vi "read_voltage0.vi"(1 "Channel":i32 min=0 max=15) -> (0 "Voltage":dbl)   [LabVIEW 2011]
uses:
  globals.vi
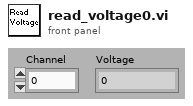
[diagram p1: front panel]
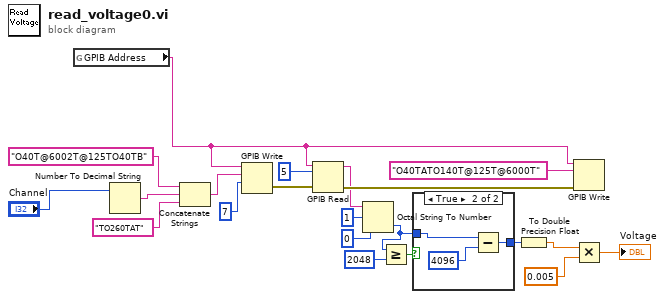
[diagram p0: block diagram]
diagram:
  n1 = global read "globals.vi" "GPIB Address"() -> (w2:string)
  n2 = Number To Decimal String(number="Channel") -> (decimal integer string=w8:string)  [unwired: 1 out]
  n3 = Concatenate Strings("O40T@6002T@125TO40TB" ("data"), w8, "TO260TAT" ("string")) -> (w7:string)
  n4 = GPIB Write(0:w2, 1:w7, 2:i16 7 ("mode (0)")) -> (6:w21:errorcluster)  [unwired: 1 in, 2 out]
  n5 = GPIB Read(0:w2, 1:5 ("byte count"), 3:w21) -> (5:w17:string, 7:w20:errorcluster)  [unwired: 3 out]
  n6 = Octal String To Number(2:0 ("default (0 U32)"), 3:1 ("offset"), 4:w17) -> (0:w11:i32)  [unwired: 1 out]
  n7 = Greater Or Equal?(x=w11, y=2048) -> (x >= y?=w12:bool)
  n8 = case shown="True" w12 {
    tunnel: w11 -> [w22 w23]
    tunnel: [w22 w25] -> w10
    frame False {
    }
    frame True {
      n9 = Subtract(x=w23, y=4096 ("x")) -> (x-y=w25:i32)
    }
  }
  n10 = To Double Precision Float(number=w10) -> (double precision float=w16:dbl)
  n11 = GPIB Write(0:w2, 1:"O40TATO140T@125T@6000T" ("data"), 3:w20) -> ()  [unwired: 4 out]
  n12 = Multiply(x=w16, y=0.005) -> (x*y=→"Voltage":dbl)
